vi "探头窗口-8.vi"() -> ()   [LabVIEW 2017]
panel:
  in  "更新数据":T1
  in  "停止信号":bool=TRUE
  out "更新数据？":bool=TRUE
  out "引用-切回列表模式？":refnum<vi>
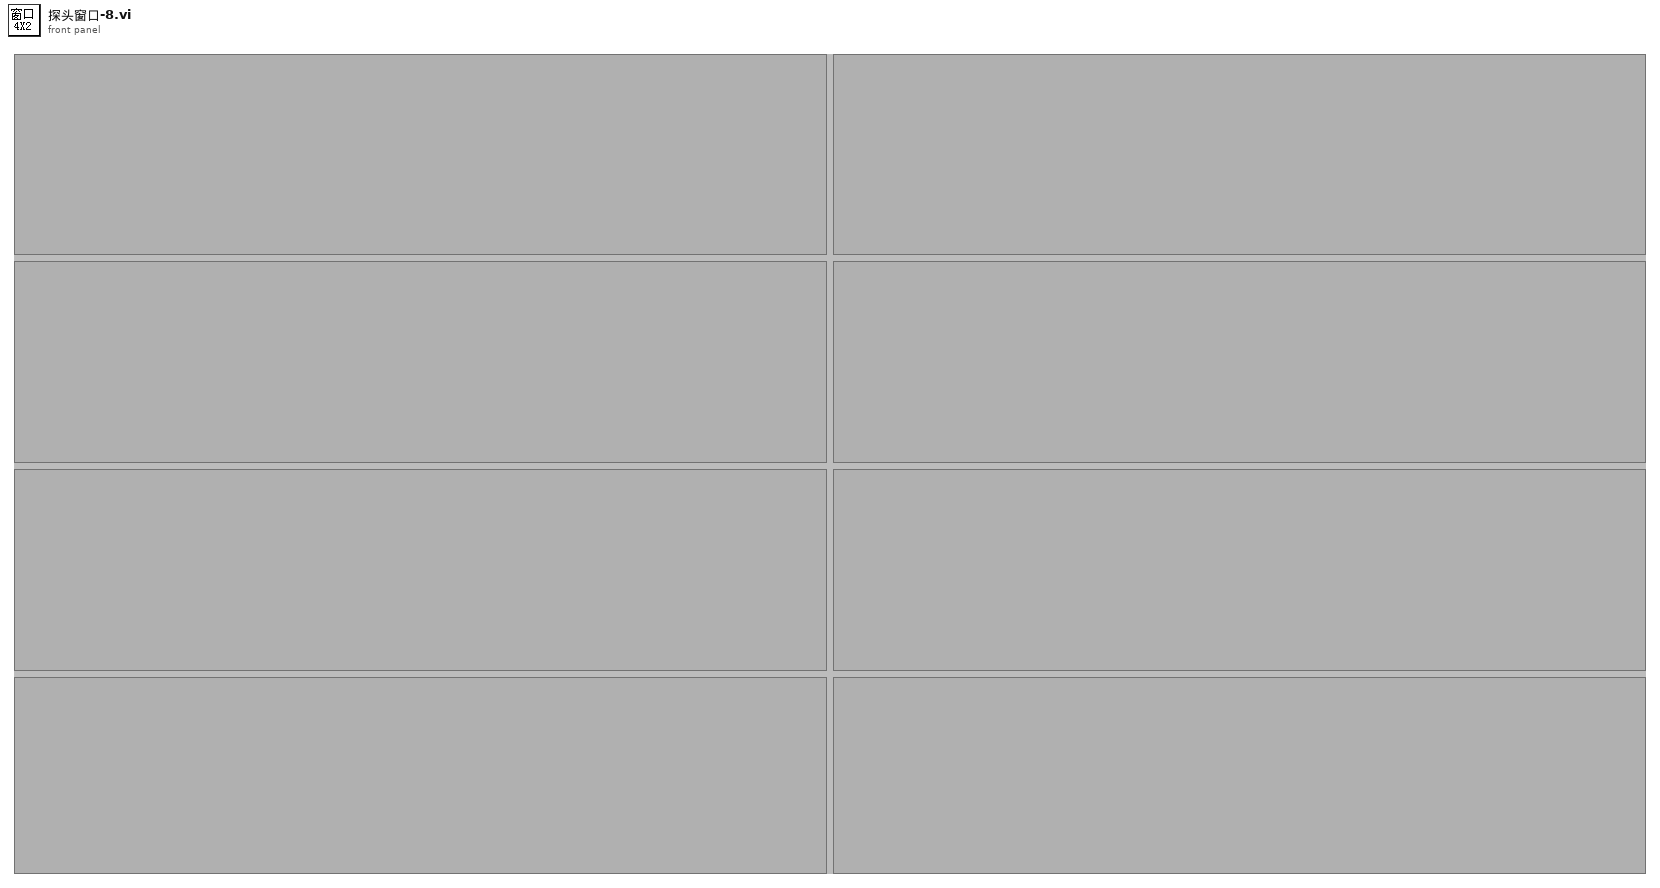
[diagram p1: front panel]
types:
  T1 = cluster{"探头启用状态？":bool[], "测量值":cluster{"X":timestamp, "Y":dbl}[], "限值":cluster{"限值1":dbl, "限值2":dbl, "探头限值":enum16{"一级限值", "二级限值"}}[], "报警状态":enum16{"正常", "一级报警", "二级报警", "累积报警"}[], "探头信息":string[], "累积剂量":cluster{"设备名称":string, "启用累积？":bool, "起始时间":timestamp, "累积剂量":dbl, "累积报警阈值":dbl}[]}
  T2 = cluster{"启用状态？":bool, "测量值":cluster{"X":timestamp, "Y":dbl}, "限值簇":cluster{"限值1":dbl, "限值2":dbl, "探头限值":enum16{"一级限值", "二级限值"}}, "报警状态":enum16{"正常", "一级报警", "二级报警", "累积报警"}, "探头信息":string, "探头地址":i32, "累积剂量":cluster{"设备名称":string, "启用累积？":bool, "起始时间":timestamp, "累积剂量":dbl, "累积报警阈值":dbl}}
  T3 = cluster{"限值1":dbl, "限值2":dbl, "探头限值":enum16{"一级限值", "二级限值"}}
  T4 = cluster{"限值1":dbl, "限值2":dbl, "探头限值":enum16{"一级限值", "二级限值"}}[]
  T5 = cluster{"设备名称":string, "启用累积？":bool, "起始时间":timestamp, "累积剂量":dbl, "累积报警阈值":dbl}[]
  T6 = cluster{"设备名称":string, "启用累积？":bool, "起始时间":timestamp, "累积剂量":dbl, "累积报警阈值":dbl}
  T7 = typedef "eventvkey.ctl" = enum16{"ASCII", "Enter", "Return", "Shift", "Ctrl", "Alt", "Cmd", "Opt", "Caps", "NumLock", "Clear", "Break", "Up", "Down", "Left", "Right", "Insert", "Delete", "Home", "End", "PageUp", "PageDown", "Escape", "Help", "Pause", "ScrollLock", "F1", "F2", "F3", "F4", "F5", "F6", "F7", "F8", "F9", "F10", "F11", "F12", "F13", "F14", "F15", "F16", "F17", "F18", "F19", "F20", "F21", "F22", "F23", "F24", "Play", "VolumeUp", "VolumeDown", "Mute", "Two Byte Char"}
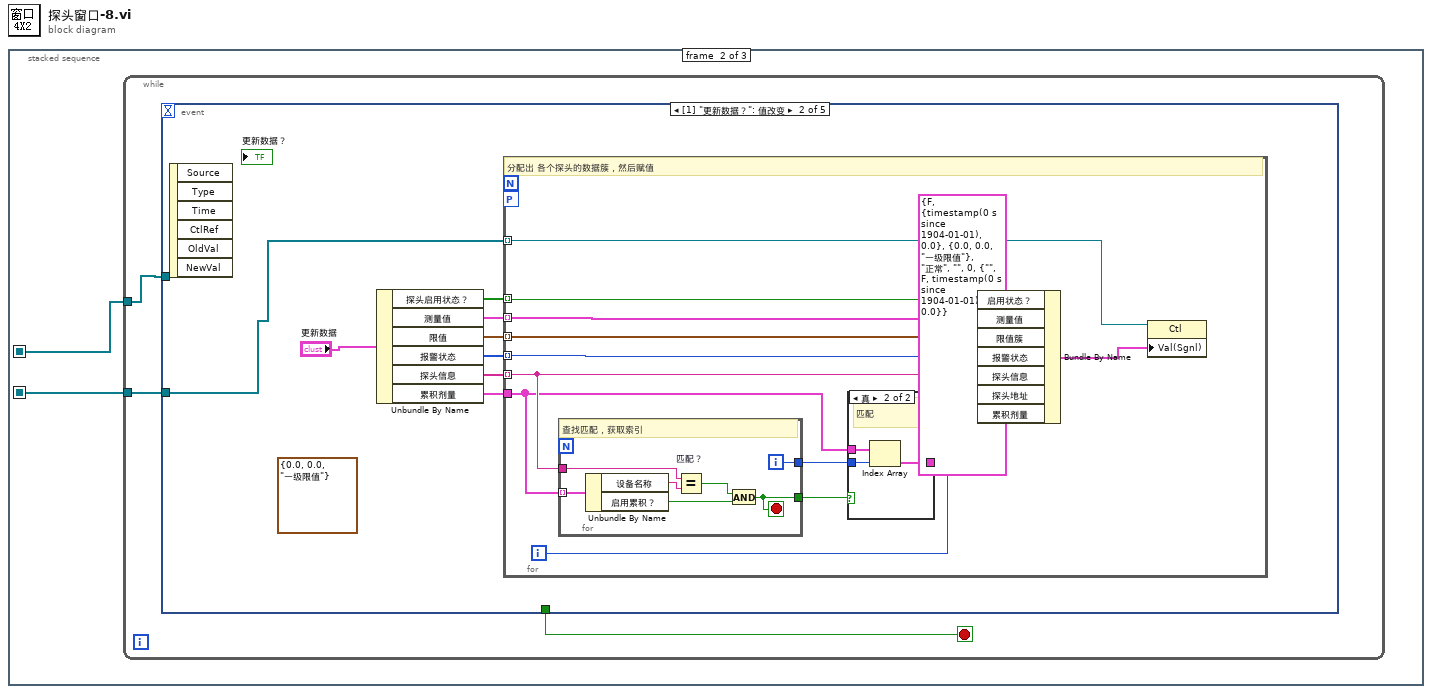
[diagram p0: block diagram]
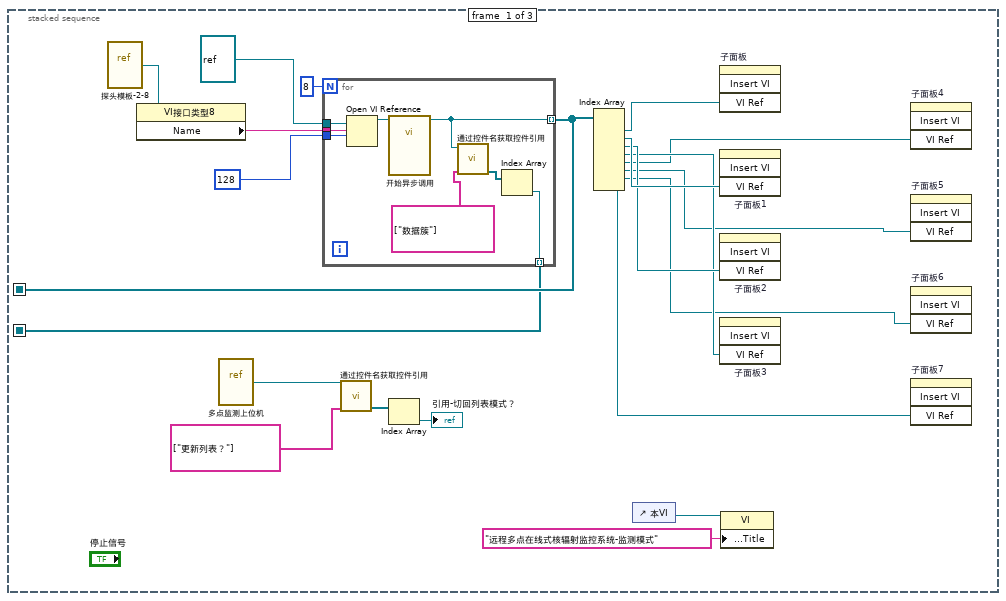
[diagram p2: hidden frame]
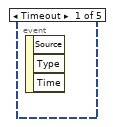
[diagram p3: hidden frame]
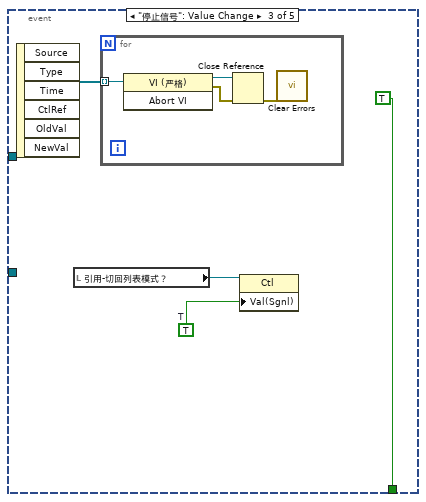
[diagram p5: hidden frame]
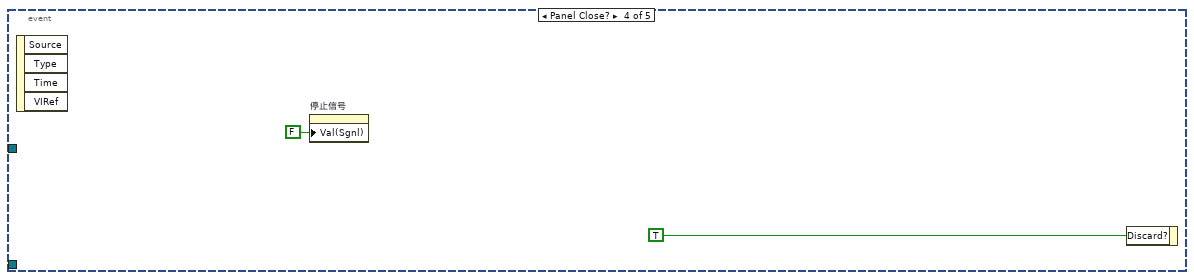
[diagram p6: hidden frame]
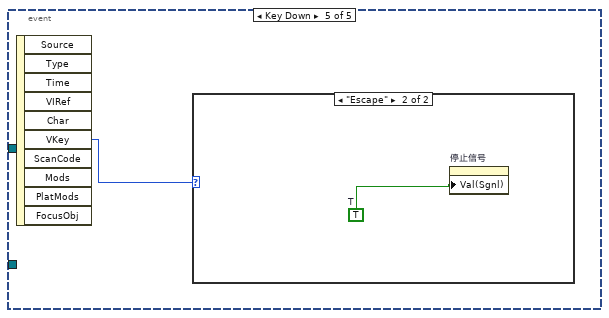
[diagram p7: hidden frame]
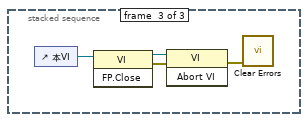
[diagram p9: hidden frame]
diagram:
  n1 = stacked-sequence {
    seq-local: [w17 _ _] -> [_ w31 _]
    seq-local: [w15 _ _] -> [_ w30 _]
    frame #0 {
      n2 = vi-ref "探头模板-2-8.vi"() -> (w21:refnum<vi>)
      n3 = property class="VI接口类型8"(reference=w21) -> ("Name"=w20:string)  [unwired: 1 in, 2 out]
      n4 = vi-ref "多点监测上位机.vi"() -> (w3:refnum<vi>)
      n5 = for {
        N: 8 -> [_]
        tunnel: w20 -> [w29]
        tunnel: 128 ("选项") -> [w28]
        tunnel: refnum<vi> refnum ("类型说明符VI引用句柄（仅用于类型）") -> [w27]
        tunnel: [w22] -> w17 mode=indexing
        tunnel: [w23] -> w15 mode=indexing
        n6 = Open VI Reference(type specifier VI Refnum (for type only)=w27, vi path=w29, options=w28) -> (vi reference=w24:refnum<vi>)  [unwired: 3 in, 1 out]
        n7 = call-by-ref "开始异步调用"(reference=w24) -> (reference out=w22:refnum<vi>)  [unwired: 13 in, 1 out]
        n8 = call "通过控件名获取控件引用.vi"("控件名数组"=string[] ["数据簇"], "VI引用"=w22) -> ("控件引用输出"=w26:refnum<vi>[])  [unwired: 7 in, 2 out]
        n9 = Index Array(array=w26) -> (element=w23:refnum<vi>)  [unwired: 1 in]
      }
      n10 = call "通过控件名获取控件引用.vi"("控件名数组"=string[] ["更新列表？"], "VI引用"=w3) -> ("控件引用输出"=w5:refnum<vi>[])  [unwired: 7 in, 2 out]
      n11 = Index Array(array=w5) -> (element=→"引用-切回列表模式？":refnum<vi>)  [unwired: 1 in]
      n12 = Index Array(array=w17) -> (element #1=w14:refnum<vi>, element #2=w13:refnum<vi>, element #3=w12:refnum<vi>, element #4=w11:refnum<vi>, element #5=w10:refnum<vi>, element #6=w9:refnum<vi>, element #7=w8:refnum<vi>, element #8=w7:refnum<vi>)  [unwired: 8 in]
      n13 = control-ref of="本VI"() -> (w2:refnum<vi>)
      n14 = invoke on="子面板" class="SubPnl" method="Insert VI"("VI Ref"=w14) -> ()  [unwired: 3 in, 4 out]
      n15 = invoke on="子面板1" class="SubPnl" method="Insert VI"("VI Ref"=w13) -> ()  [unwired: 3 in, 4 out]
      n16 = invoke on="子面板2" class="SubPnl" method="Insert VI"("VI Ref"=w12) -> ()  [unwired: 3 in, 4 out]
      n17 = invoke on="子面板3" class="SubPnl" method="Insert VI"("VI Ref"=w11) -> ()  [unwired: 3 in, 4 out]
      n18 = property class="VI"(reference=w2, "Front Panel.Title"="远程多点在线式核辐射监控系统-监测模式" ("前面板窗口:标题")) -> ()  [unwired: 1 in, 2 out]
      n19 = invoke on="子面板4" class="SubPnl" method="Insert VI"("VI Ref"=w10) -> ()  [unwired: 3 in, 4 out]
      n20 = invoke on="子面板5" class="SubPnl" method="Insert VI"("VI Ref"=w9) -> ()  [unwired: 3 in, 4 out]
      n21 = invoke on="子面板6" class="SubPnl" method="Insert VI"("VI Ref"=w8) -> ()  [unwired: 3 in, 4 out]
      n22 = invoke on="子面板7" class="SubPnl" method="Insert VI"("VI Ref"=w7) -> ()  [unwired: 3 in, 4 out]
    }
    frame #1 {
      n23 = while {
        tunnel: w31 -> [w33]
        tunnel: w30 -> [w32]
        stop <- w34 stop-if-true
        n24 = event shown="[1] \"更新数据？\": 值改变" {
          selector: _ -> [_ _ _ _ _]
          dyn-events: _ -> [_ _ _ _ _]
          timeout: _ -> [_ _ _ _ _]
          tunnel: [_ _ TRUE ("放弃？") _ _] -> w34
          tunnel: w33 -> [_ _ w68 _ _]
          tunnel: w32 -> [_ w35 _ _ _]
          event Timeout {
            n25 = event-data() -> ()  [unwired: 1 in, 3 out]
          }
          event "更新数据？": Value Change {
            (unwired) T3 {"限值1"=0.0, "限值2"=0.0, "探头限值"=enum."一级限值"} ("探头限值簇")
            n26 = event-data() -> ()  [unwired: 1 in, 6 out]
            n27 = Unbundle By Name("更新数据") -> ("探头启用状态？"=w36:bool[], "测量值"=w37:cluster{"X":timestamp, "Y":dbl}[], "限值"=w38:T4, "报警状态"=w39:enum16{"正常", "一级报警", "二级报警", "累积报警"}[], "探头信息"=w40:string[], "累积剂量"=w41:T5)
            n28 = for {
              tunnel: w36 -> [w55] mode=indexing
              tunnel: w37 -> [w54] mode=indexing
              tunnel: w38 -> [w53] mode=indexing
              tunnel: w39 -> [w52] mode=indexing
              tunnel: w40 -> [w47] mode=indexing
              workers-P: _ -> [_]
              tunnel: w35 -> [w50] mode=indexing
              tunnel: w41 -> [w46]
              i -> [w48]
              # "分配出 各个探头的数据簇，然后赋值"
              n29 = for {
                tunnel: w46 -> [w65] mode=indexing
                tunnel: w47 -> [w63]
                tunnel: [w60] -> w45
                tunnel: [w59] -> w44
                i -> [w60]
                stop <- w59 stop-if-true
                # "查找匹配，获取索引"
                n30 = Unbundle By Name(w65) -> ("设备名称"=w64:string, "启用累积？"=w61:bool)
                n31 = Equal? "匹配？"(x=w63, y=w64) -> (x = y?=w62:bool)
                n32 = And(x=w62, y=w61) -> (x .and. y?=w59:bool)
              }
              n33 = case shown="真" w44 {
                tunnel: w46 -> [_ w58]
                tunnel: w45 -> [_ w57]
                tunnel: [_ w56] -> w43
                frame False {
                  # "不匹配"
                }
                frame True {
                  # "匹配"
                  n34 = Index Array(array=w58, index=w57) -> (element=w56:T6)
                }
              }
              n35 = Bundle By Name(cluster=T2 {"启用状态？"=FALSE, "测量值"={"X"=timestamp(0 s since 1904-01-01), "Y"=0.0}, "限值簇"={"限值1"=0.0, "限值2"=0.0, "探头限值"=enum."一级限值"}, "报警状态"=enum."正常", "探头信息"="", "探头地址"=0, "累积剂量"={"设备名称"="", "启用累积？"=FALSE, "起始时间"=timestamp(0 s since 1904-01-01), "累积剂量"=0.0, "累积报警阈值"=0.0}} ("输出簇"), "启用状态？"=w55, "测量值"=w54, "限值簇"=w53, "报警状态"=w52, "探头信息"=w47, "探头地址"=w48, "累积剂量"=w43) -> (w49:T2)
              n36 = property class="Ctl"(reference=w50, "Val(Sgnl)"=w49) -> ()  [unwired: 1 in, 2 out]
            }
          }
          event "停止信号": Value Change {
            w67 = TRUE  # T
            n37 = event-data() -> ()  [unwired: 1 in, 6 out]
            n38 = local read "引用-切回列表模式？"() -> (w66:refnum<vi>)
            n39 = for {
              tunnel: w68 -> [w73] mode=indexing
              n40 = invoke class="VI (严格)" method="Abort VI"(reference=w73) -> (reference out=w71:refnum<vi>, error out=w72:errorcluster)  [unwired: 2 in, 1 out]
              n41 = Close Reference(reference=w71, error in (no error)=w72) -> (error out=w70:errorcluster)
              n42 = call <vilib>:"Clear Errors.vi"("error in (no error)"=w70) -> ()  [unwired: 5 in, 2 out]
            }
            n43 = property class="Ctl"(reference=w66, "Val(Sgnl)"=w67) -> ()  [unwired: 1 in, 2 out]
          }
          event Panel Close? {
            n44 = event-data() -> ()  [unwired: 1 in, 4 out]
            n45 = property on="停止信号" class="Bool (严格)"("Val(Sgnl)"=FALSE ("值(信号)")) -> ()  [unwired: 2 in, 2 out]
            n46 = event-data("Discard?"=TRUE ("放弃？")) -> ()  [unwired: 1 in, 1 out]
          }
          event Key Down {
            n47 = event-data() -> ("VKey"=w76:T7)  [unwired: 1 in, 9 out]
            n48 = case shown="\"Escape\"" w76 {
              frame "ASCII", Default {
              }
              frame "Escape" {
                w77 = TRUE  # T
                n49 = property on="停止信号" class="Bool (严格)"("Val(Sgnl)"=w77) -> ()  [unwired: 2 in, 2 out]
              }
            }
          }
        }
      }
    }
    frame #2 {
      n50 = control-ref of="本VI"() -> (w81:refnum<vi>)
      n51 = invoke class="VI" method="FP.Close"(reference=w81) -> (reference out=w80:refnum<vi>, error out=w79:errorcluster)  [unwired: 2 in, 1 out]
      n52 = invoke class="VI" method="Abort VI"(reference=w80, error in=w79) -> (error out=w78:errorcluster)  [unwired: 1 in, 2 out]
      n53 = call <vilib>:"Clear Errors.vi"("error in (no error)"=w78) -> ()  [unwired: 5 in, 2 out]
    }
  }
